vi "1_Main.vi"() -> ()   [LabVIEW 2014]
uses:
  <vilib>/Platform/TimedLoop/XDataNode/timing_clust.ctl
  <vilib>/Platform/TimedLoop/XDataNode/nitl_modes.ctl
  <vilib>/Platform/TimedLoop/XDataNode/wakeup.ctl
  <vilib>/myRIO/Instrument Drivers/Onboard IO/UART/typedef/VISA Configuration.ctl
  <vilib>/myRIO/Instrument Drivers/Onboard IO/DIO/typedefs/DIO Reference.ctl
  <vilib>/myRIO/Common/Instrument Driver Framework/Utilities/typedefs/myRIO Generic Hardware Reference.ctl
  <vilib>/myRIO/Common/Instrument Driver Framework/Utilities/typedefs/Hardware Version Enum.ctl
  <vilib>/myRIO/Common/Instrument Driver Framework/Utilities/typedefs/myRIO v1.0 Reference.ctl
  <vilib>/myRIO/Common/Instrument Driver Framework/Utilities/typedefs/Generic FPGA Reference.ctl
  <vilib>/myRIO/Common/Instrument Driver Framework/myRIO v1.0/DIO/typedefs/DIO Channels List.ctl
  <vilib>/myRIO/Common/Instrument Driver Framework/myRIO v1.0/DIO/typedefs/DIO Channels Enum.ctl
  <vilib>/userdefined/High Color/nirio_resource_hc.ctl
  <vilib>/myRIO/Instrument Drivers/Onboard Devices/Accelerometer/typedefs/Accelerometer Reference.ctl
  <vilib>/myRIO/Common/Instrument Driver Framework/myRIO v1.0/Accelerometer/typedefs/Accelerometer Channels List.ctl
  <vilib>/myRIO/Common/Instrument Driver Framework/myRIO v1.0/Accelerometer/typedefs/Accelerometer Channels Enum.ctl
  <vilib>/myRIO/Common/Instrument Driver Framework/Utilities/vis/Is FPGA Ref Available.vi
  <vilib>/myRIO/Common/Instrument Driver Framework/myRIO v1.0/DIO/vis/myRIO v1.1 Open DIO.vi
  <vilib>/myRIO/Instrument Drivers/Onboard IO/DIO/vis/Write.vi
  <vilib>/myRIO/Common/Instrument Driver Framework/myRIO v1.0/Accelerometer/vis/myRIO v1.1 Open Accelerometer.vi
  <vilib>/myRIO/Instrument Drivers/Onboard Devices/Accelerometer/vis/Read.vi
  <vilib>/myRIO/Common/Instrument Driver Framework/Utilities/vis/Validate Channels.vi
  <vilib>/myRIO/Common/Instrument Driver Framework/myRIO v1.0/DIO/vis/myRIO v1.0 Reserve DIO.vi
  <vilib>/myRIO/Common/Instrument Driver Framework/myRIO v1.0/Accelerometer/vis/myRIO v1.0 Reserve Accelerometer.vi
  <vilib>/myRIO/Common/Instrument Driver Framework/myRIO v1.0/UART/vis/myRIO v1.0 Close UART.vi
  <vilib>/myRIO/Common/Instrument Driver Framework/myRIO v1.0/Resource Manager/vis/myRIO v1.0 Reserve Channel List.vi
  <vilib>/myRIO/Common/Instrument Driver Framework/myRIO v1.0/DIO/vis/myRIO v1.0 Build MUX Configuration DIO.vi
  <vilib>/myRIO/Common/Instrument Driver Framework/myRIO v1.0/Accelerometer/vis/myRIO v1.0 Build MUX Configuration Accelerometer.vi
  <vilib>/myRIO/Common/Instrument Driver Framework/myRIO v1.0/Resource Manager/vis/myRIO v1.0 Reserve Channel.vi
  <vilib>/myRIO/Common/Instrument Driver Framework/myRIO v1.0/Resource Manager/vis/myRIO v1.0 Unreserve Channel.vi
  <vilib>/myRIO/Common/Instrument Driver Framework/myRIO v1.0/Resource Manager/vis/myRIO v1.0 Create Configuration List.vi
  <vilib>/myRIO/Common/Instrument Driver Framework/myRIO v1.0/Resource Manager/vis/myRIO v1.0 Build Mutex Name.vi
  <vilib>/Instr/_visa.llb/VISA Configure Serial Port (Instr).vi
  <vilib>/Utility/VariantDataType/GetNumericInfo.vi
  <vilib>/Utility/error.llb/Error Cluster From Error Code.vi
  <vilib>/myRIO/Common/Instrument Driver Framework/myRIO v1.0/myRIO v1.1 Open.vi
  <vilib>/myRIO/Common/Instrument Driver Framework/Utilities/vis/IO Manager.vi
  <vilib>/myRIO/Common/Instrument Driver Framework/Utilities/vis/Configuration Manager.vi
  <vilib>/myRIO/Common/Instrument Driver Framework/myRIO v1.0/Resource Manager/vis/myRIO v1.0 Configure IO.vi
  <vilib>/myRIO/Common/Instrument Driver Framework/myRIO v1.0/myRIO v1.0 Close.vi
  <vilib>/myRIO/Common/Instrument Driver Framework/myRIO v1.0/DIO/vis/myRIO v1.0 Write DIO.vi
  <vilib>/myRIO/Common/Instrument Driver Framework/myRIO v1.0/Accelerometer/vis/myRIO v1.0 Get Scaling Constant Accelerometer.vi
  <vilib>/myRIO/Common/Instrument Driver Framework/myRIO v1.0/Accelerometer/vis/myRIO v1.0 Read Accelerometer.vi
  <vilib>/myRIO/Common/Instrument Driver Framework/Utilities/vis/FPGA Ref Manager.vi
  <vilib>/myRIO/Common/Instrument Driver Framework/myRIO v1.0/myRIO v1.0 Reset FPGA.vi
  <vilib>/myRIO/Common/Instrument Driver Framework/myRIO v1.0/IRQ/vis/myRIO v1.0 IRQ Info FGV.vi
  <vilib>/myRIO/Common/Instrument Driver Framework/myRIO v1.0/IRQ/vis/myRIO v1.0 Timer IRQ Info FGV.vi
  <vilib>/myRIO/Common/Instrument Driver Framework/myRIO v1.0/IRQ/vis/myRIO v1.0 ISR Agent.vi
  <vilib>/myRIO/Express VI/Onboard IO/UART/UART Express VI.xnode
  <vilib>/platform/TimedLoop/XDataNode/XDataNode.xnode
  <vilib>/myRIO/Express VI/Onboard Devices/LED/LED Express VI.xnode
  <vilib>/myRIO/Instrument Drivers/Onboard IO/DIO/vis/myRIO DIO Open.xnode
  <vilib>/myRIO/Express VI/Onboard Devices/Accelerometer/Accelerometer Express VI.xnode
  <vilib>/myRIO/Instrument Drivers/Onboard Devices/Accelerometer/vis/myRIO Accelerometer Open.xnode
  <vilib>/myRIO/Instrument Drivers/Utilities/Utilities.lvlib
  <vilib>/myRIO/Instrument Drivers/Onboard Devices/Accelerometer/Accelerometer.lvlib
  <vilib>/myRIO/Instrument Drivers/Onboard IO/DIO/DIO.lvlib
  <vilib>/myRIO/Instrument Drivers/Onboard IO/UART/UART.lvlib
  <vilib>/Platform/TimedLoop/XDataNode/XDNodeRunTimeDep.lvlib
panel:
  out "Measured Angle":dbl
  out "Simulation Angle":dbl
  out "Receive Distance":bool
  out "Velocity Display":dbl(graph)
  out "Data File Path":path=path "c:/ni-rt/startup/11_25_14_03:39 AM.csv"
  out "Read Finished Late?":bool
  out "Velocity (cm/s)":dbl(slide) scale=0.0..100.0
  out "match substring":string
  out "Distance (cm)":dbl
  in  "Simulation":bool=TRUE
  in  "PS 14":bool caption="1"
  in  "PS 13":bool caption="1"
  in  "PS 12":bool caption="1"
  in  "PS 11":bool caption="1"
  in  "PS 10":bool caption="1"
  in  "PS 9":bool caption="1"
  in  "PS 8":bool caption="1"
  in  "PS 7":bool caption="1"
  in  "PS 6":bool caption="1"
  in  "PS 5":bool caption="1"
  in  "PS 4":bool caption="1"
  in  "PS 3":bool caption="1"
  in  "PS 2":bool caption="1"
  in  "PS 1":bool caption="1"
  in  "Arm Leg Angle Ratio":dbl(slide)=0.9696969696969697 scale=0.0..2.0
  in  "Ground":dbl(slide)=400.00000000000006 scale=0.0..450.0
  in  "Horizontal Center":dbl(slide)=395.95959595959596 scale=0.0..800.0
  out "Characters Read":string
  out "Mannequin Motion":picture
  out "Joint A":dbl(knob)=7.460836761961528 scale=40.0..-40.0 scale format="%#.1f"
  in  "Scale Factor":dbl(slide)=0.5707070707070707 scale=0.5..1.0
  in  "LED3":bool
  in  "LED2":bool
  in  "LED1":bool
  in  "LED0":bool
  out "Acceleration":T1(graph)={"X-Axis"=0.0625, "Y-Axis"=0.109375, "Z-Axis"=1.0}
  out "error out":errorcluster
  in  "Stop Button":bool
  # "Overview: The myRIO Project template acquires acceleration data from the onboard accelerometer and displays the changes of acceleration values in a waveform chart.\nInstructions:\n1. Check the myRIO target IP Address in the project and make sure the target IP Address is correct. \n2. Run the VI."
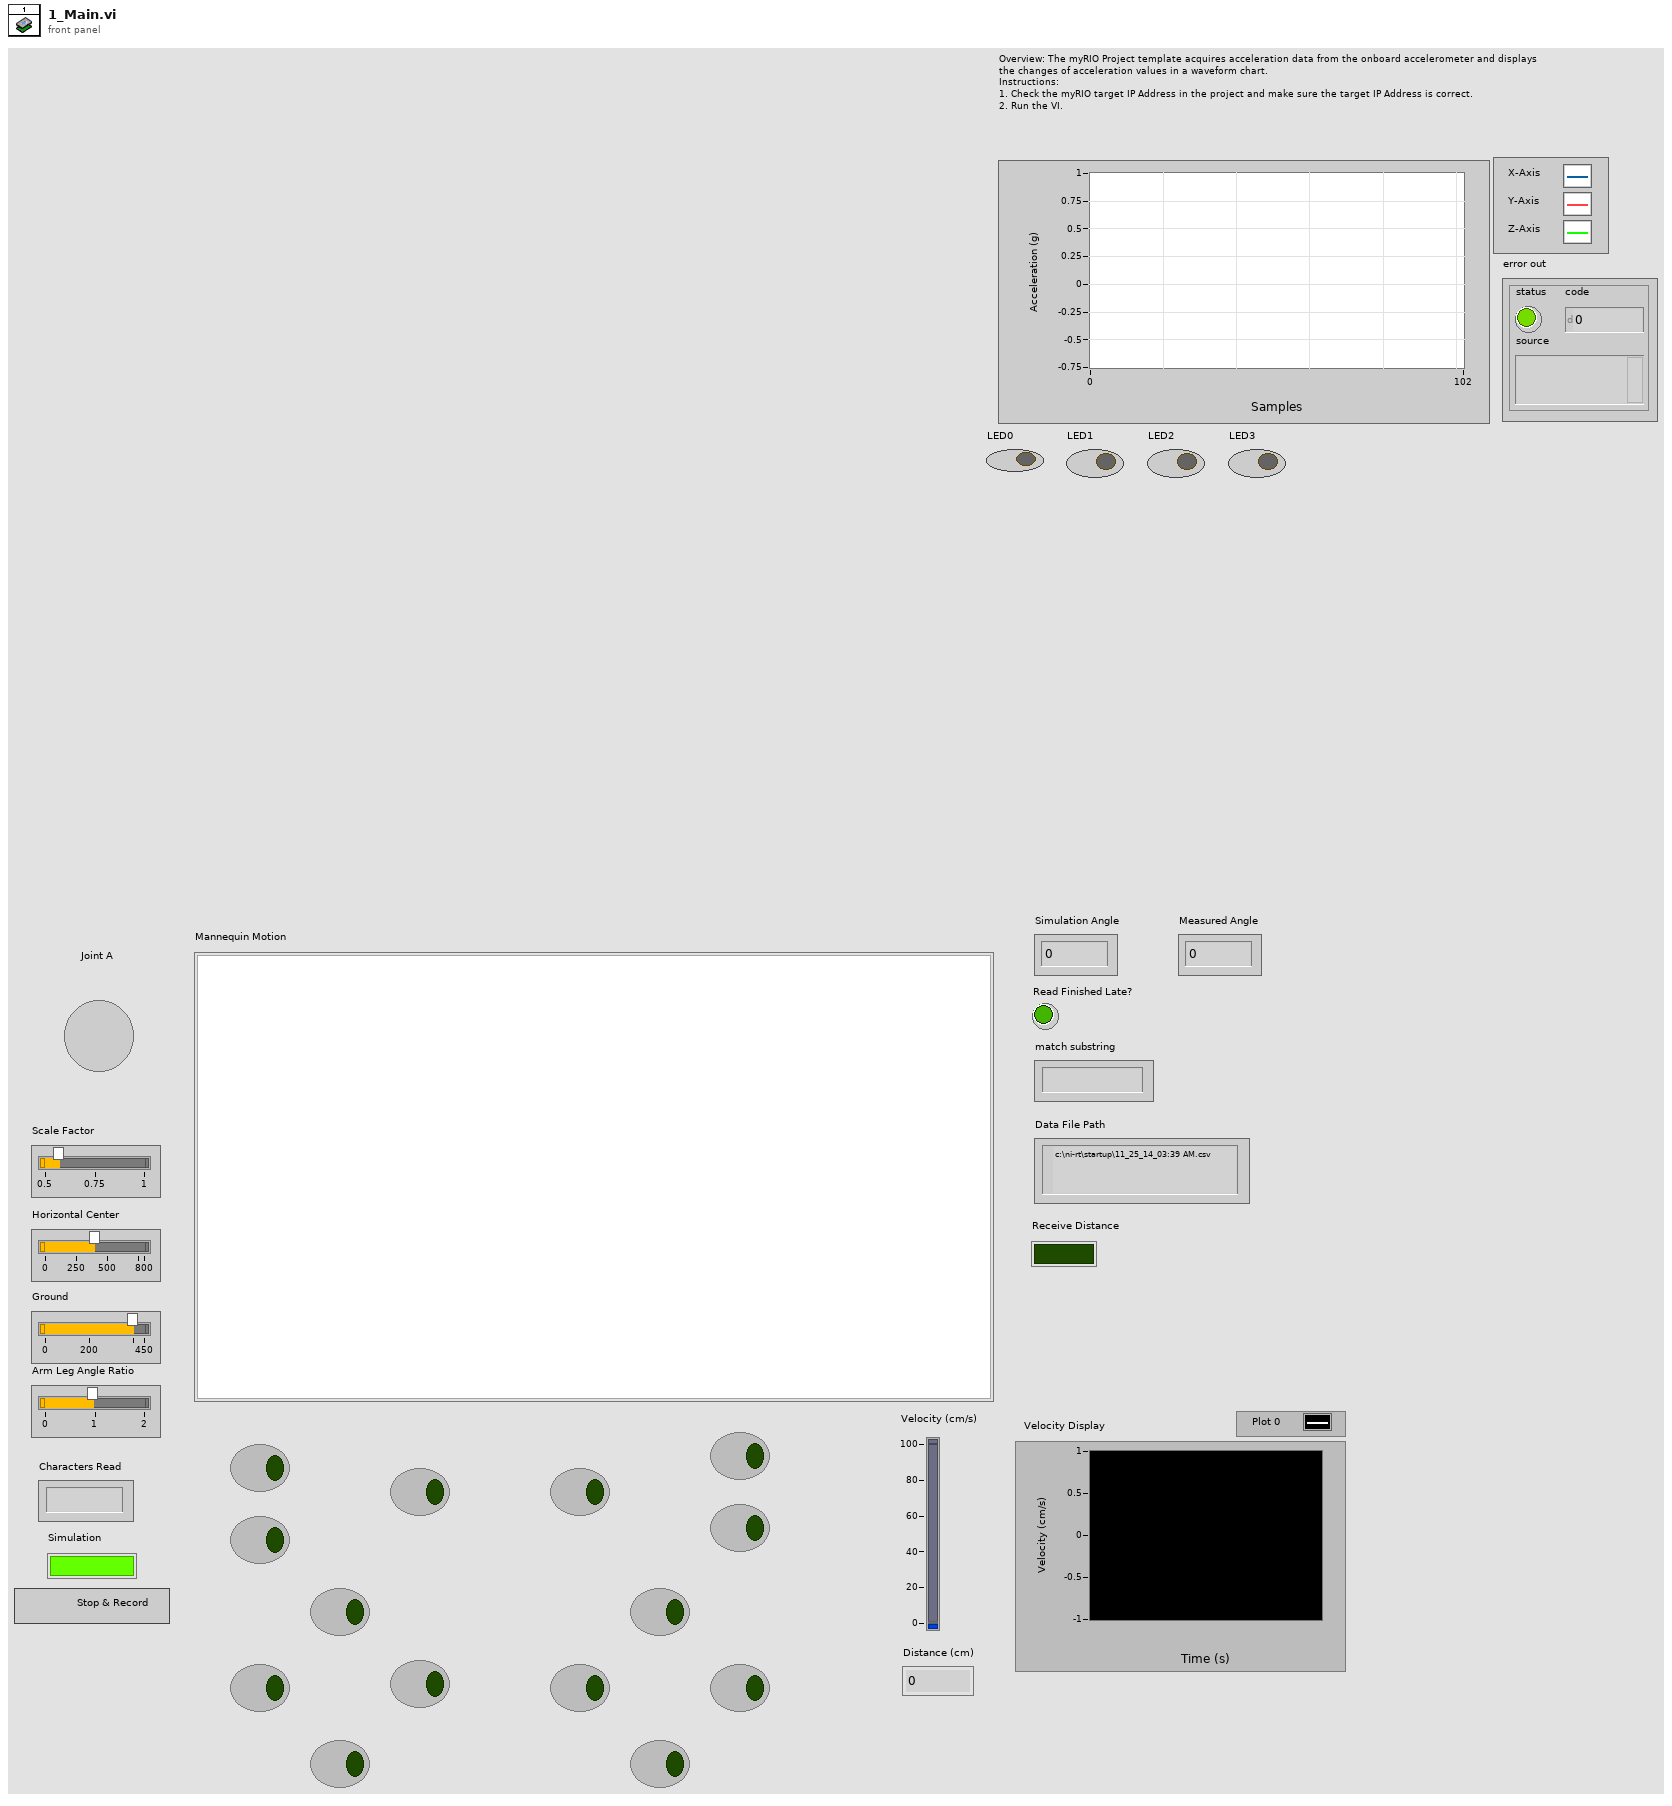
[diagram p1: front panel]
types:
  T1 = cluster{"X-Axis":dbl, "Y-Axis":dbl, "Z-Axis":dbl}
  T2 = typedef "XDNodeRunTimeDep.lvlib/timing_clust.ctl" = cluster{"Expected End [f-1]":u64, "Actual End [f-1]":u64, "Finished Late? [f-1]":bool, "Expected End [i-1]":u64, "Actual End [i-1]":u64, "Finished Late? [i-1]":bool, "Expected Start [i]":u64, "Actual Start [i]":u64, "Expected Start [f]":u64, "Actual Start [f]":u64, "Source Name":string, "Structure Name":string, "Period":i64, "Deadline":i64, "Offset":i64, "Start":i64, "Priority":i32, "Timeout":i32, "Mode":T3, "Wakeup Reason":T4, "Error":errorcluster, "Source Type":string, "Secondary Source Type":string, "Global End Time":u64, "Global Start Time":u64, "Frame Duration":u64, "Iteration Duration":u64, "Assigned CPU":i32, "I/O Scan Engine Mode":u32}
  T3 = typedef "XDNodeRunTimeDep.lvlib/nitl_modes.ctl" = enum32{"No Change", "Process missed periods, maintain original phase", "Discard missed periods, maintain original phase", "Process missed periods, ignore original phase", "Discard missed periods, ignore original phase"}
  T4 = typedef "XDNodeRunTimeDep.lvlib/wakeup.ctl" = enum32{"Normal", "Aborted", "Asynchronous wakeup", "Timing source error", "Timed loop error", "Timeout"}
  T5 = typedef "UART.lvlib/VISA Configuration.ctl" = cluster{"baud rate (9600)":u32, "data bits (8)":u16, "parity (0:none)":enum16{"None", "Odd", "Even", "Mark", "Space"}, "stop bits (10: 1 bit)":u16, "flow control (0:none)":u16, "termination char\n(0xA = '\\n' = LF) ":u8, "Enable Termination\nChar (T)":bool, "timeout (10sec)":u32}
  T6 = cluster{"Width":u16, "Style":enum32{"Solid", "Dash", "Dot", "DashDot", "DashDotDot"}}
  T7 = cluster{"left":i16, "top":i16, "right":i16, "bottom":i16}
  T8 = typedef "DIO.lvlib/DIO Reference.ctl" = cluster{"myRIO Reference":T9, "DIO Channels List":T13}
  T9 = typedef "myRIO Generic Hardware Reference.ctl" = cluster{"myRIO Model":T10, "myRIO Hardware Reference":T11}
  T10 = typedef "Hardware Version Enum.ctl" = enum16{"Unknown", "myRIO-1900", "myRIO-1950"}
  T11 = typedef "myRIO v1.0 Reference.ctl" = cluster{"Generic FPGA Reference":T12, "Allow multiple opens":bool}
  T12 = typedef "Generic FPGA Reference.ctl" = refnum<k20>
  T13 = typedef "DIO Channels List.ctl" = T14[]
  T14 = typedef "DIO Channels Enum.ctl" = enum16{"Not Connected", "C/DIO0", "C/DIO1", "C/DIO2", "C/DIO3", "C/DIO4", "C/DIO5", "C/DIO6", "C/DIO7", "A/DIO0", "A/DIO1", "A/DIO2", "A/DIO3", "A/DIO4", "A/DIO5", "A/DIO6", "A/DIO7", "A/DIO8", "A/DIO9", "A/DIO10", "A/DIO11", "A/DIO12", "A/DIO13", "A/DIO14", "A/DIO15", "B/DIO0", "B/DIO1", "B/DIO2", "B/DIO3", "B/DIO4", "B/DIO5", "B/DIO6", "B/DIO7", "B/DIO8", "B/DIO9", "B/DIO10", "B/DIO11", "B/DIO12", "B/DIO13", "B/DIO14", "B/DIO15", "LED0", "LED1", "LED2", "LED3", "Button0"}
  T15 = typedef "nirio_resource_hc.ctl" = tag
  T16 = typedef "Accelerometer.lvlib/Accelerometer Reference.ctl" = cluster{"myRIO Reference":T9, "Accelerometer Channels List":T17, "LSB Weight":dbl}
  T17 = typedef "Accelerometer Channels List.ctl" = T18[]
  T18 = typedef "Accelerometer Channels Enum.ctl" = enum16{"Not Connected", "X-Axis", "Y-Axis", "Z-Axis"}
  T19 = enum16{"open", "replace", "create", "open or create", "replace or create", "replace or create with confirmation"}
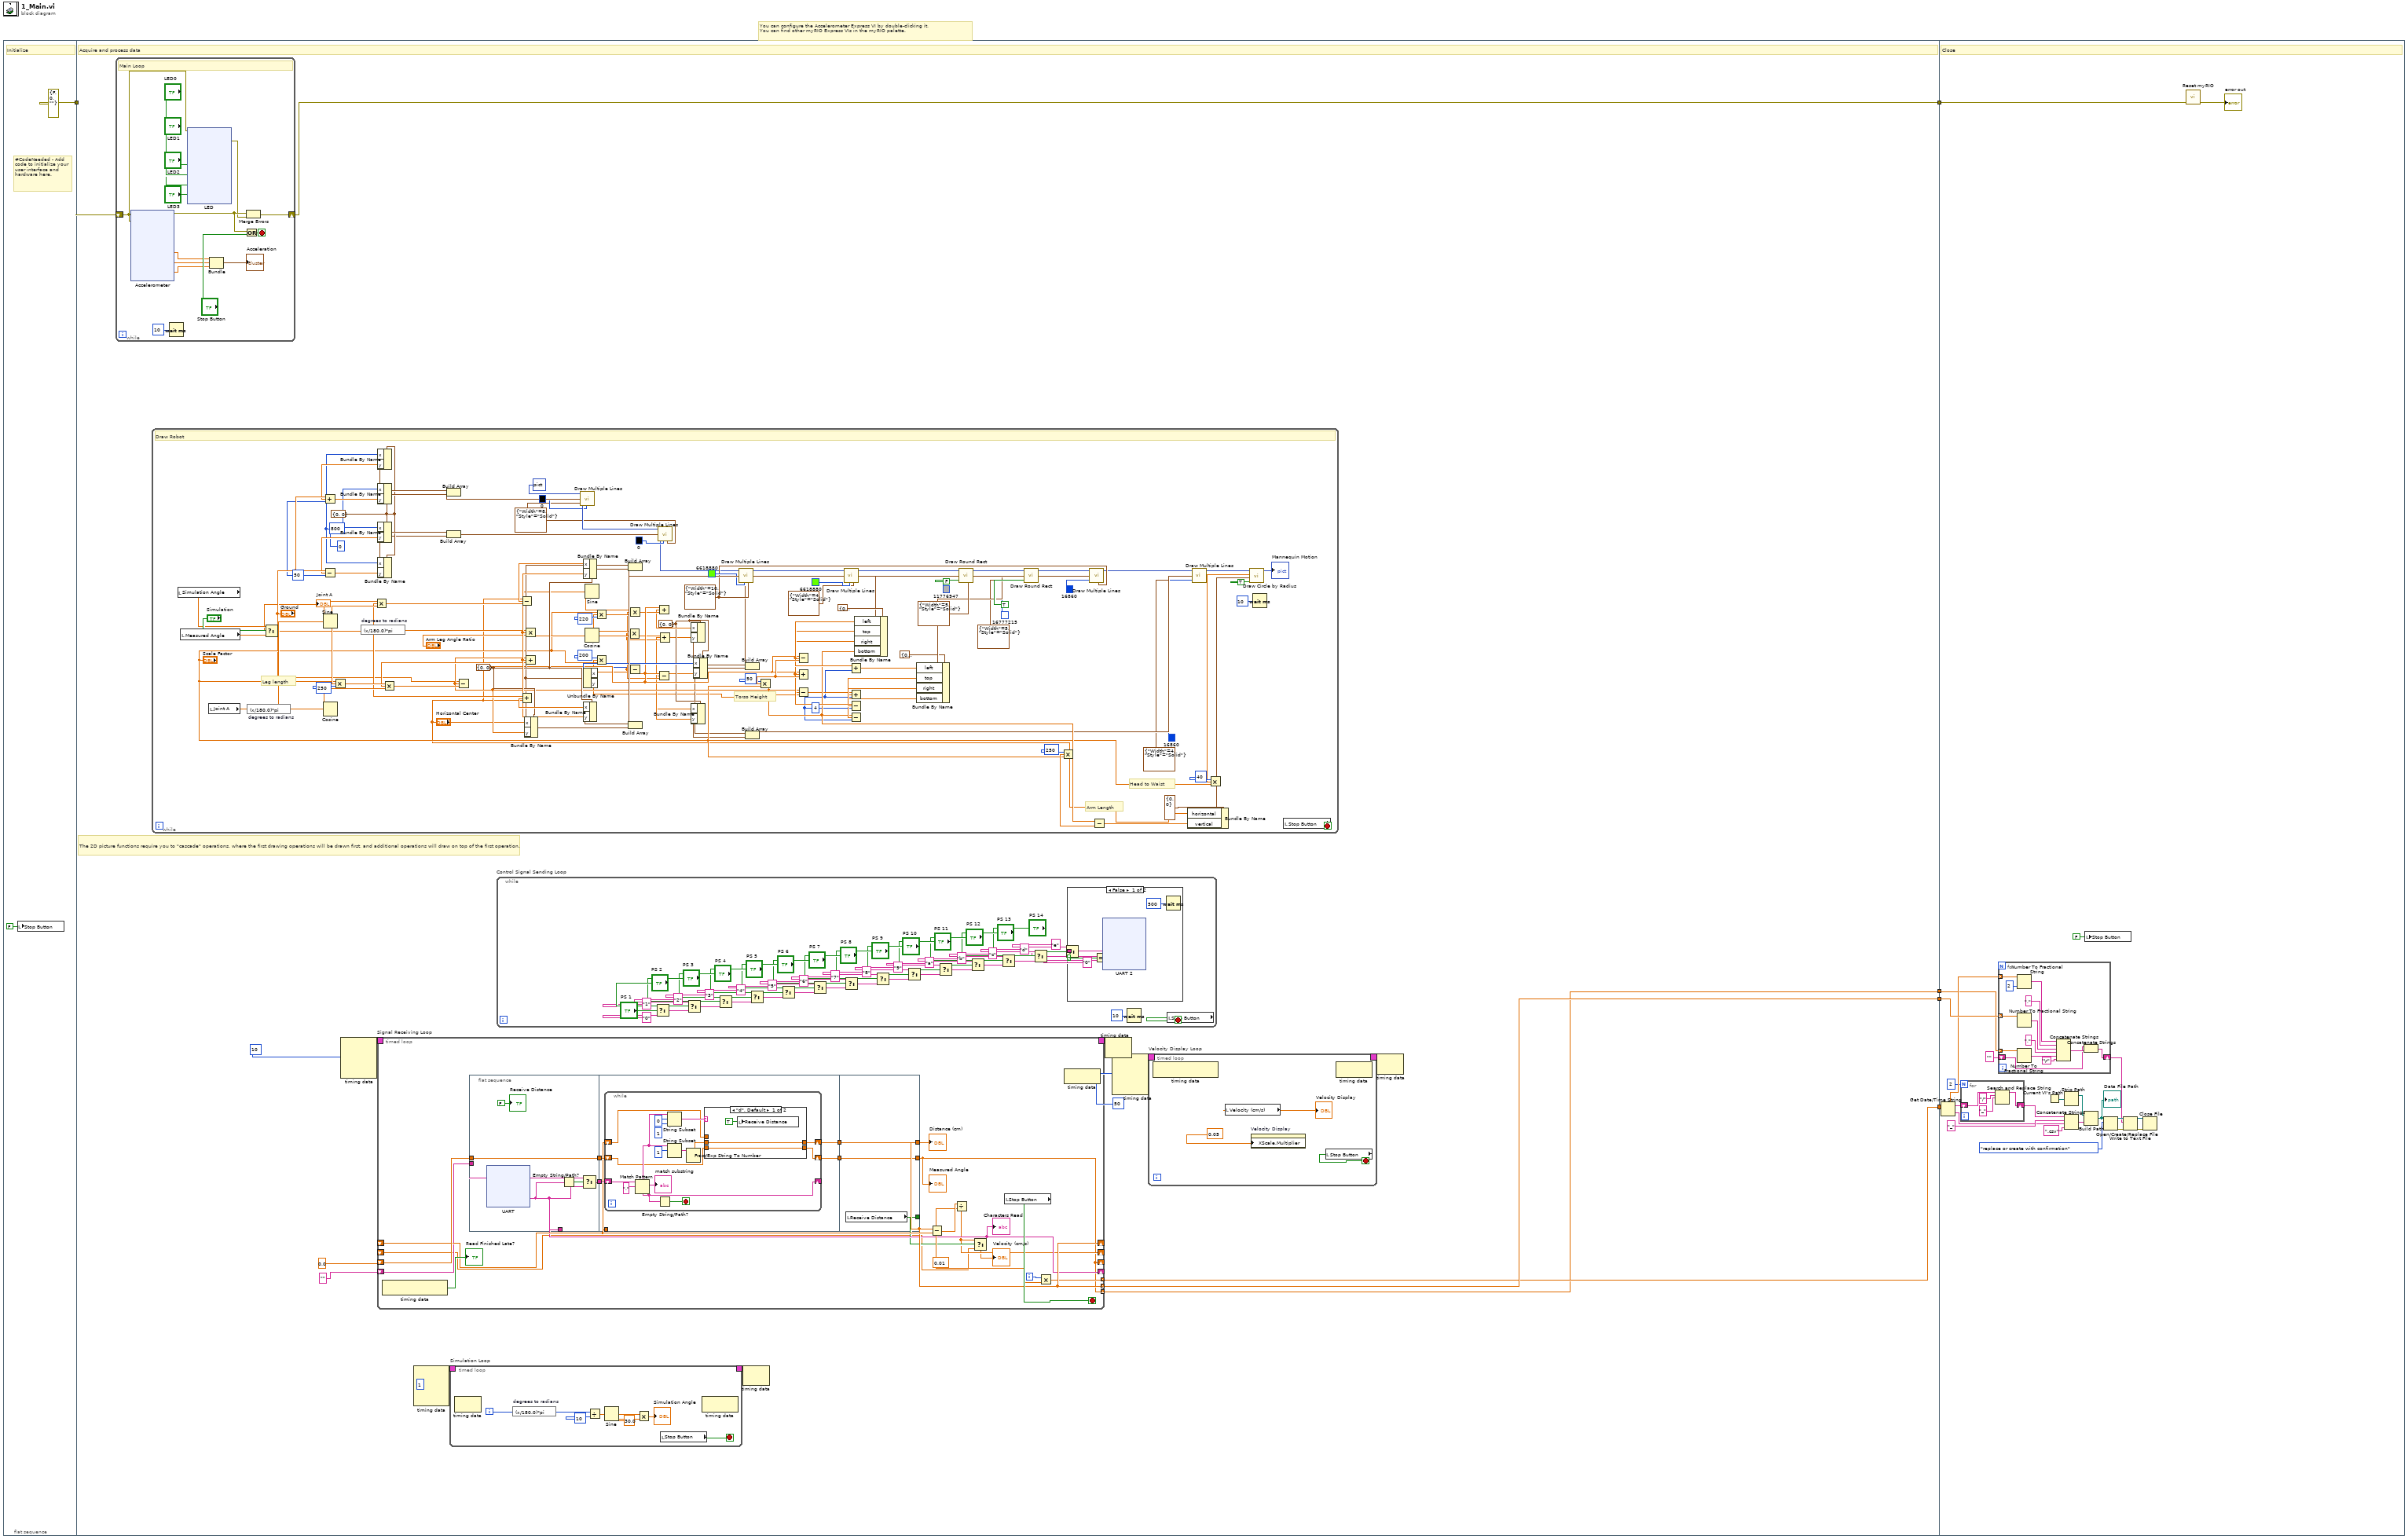
[diagram p0: block diagram]
diagram:
  # "You can configure the Accelerometer Express VI by double-clicking it.\nYou can find other myRIO Express VIs in the myRIO palette."
  n1 = flat-sequence {
    tunnel: [errorcluster {"status"=FALSE, "code"=0, "source"=""} ("error out")] -> w5
    tunnel: w5 -> [w23]
    tunnel: [w22] -> w4
    tunnel: [w16] -> w3
    tunnel: [w15] -> w2
    tunnel: [w14] -> w1
    tunnel: w4 -> [w415]
    tunnel: w3 -> [w406]
    tunnel: w2 -> [w405]
    tunnel: w1 -> [w404]
    frame #0 {
      # "#CodeNeeded - Add code to initialize your user interface and hardware here."
      # "Initialize"
      n2 = local write "Stop Button"(FALSE ("Stop Button")) -> ()
    }
    frame #1 {
      # "The 2D picture functions require you to \"cascade\" operations, where the first drawing operations will be drawn first, and additional operations will draw on top of the first operation."
      # "Acquire and process data"
      n3 = while {
        shift-right: [w301] -> w22
        shift-left: w23 -> [w302]
        stop <- w314 stop-if-true
        # "Main Loop"
        n4 = xnode "Accelerometer"("error in (no error)"=w302) -> ("X-Axis"=w311:dbl, "Y-Axis"=w310:dbl, "Z-Axis"=w309:dbl, "error out"=w304:errorcluster)
        n5 = Wait (ms)(milliseconds to wait=u32 10) -> ()  [unwired: 1 out]
        n6 = xnode "LED"("LED0"="LED0", "LED1"="LED1", "LED2"="LED2", "LED3"="LED3", "error in (no error)"=w302) -> ("error out"=w303:errorcluster)
        n7 = Bundle("X-Axis"=w311, "Y-Axis"=w310, "Z-Axis"=w309) -> (→"Acceleration":T1)  [unwired: 1 in]
        n8 = Or(x=w304, y="Stop Button") -> (x .or. y?=w314:bool)
        n9 = Merge Errors(w304, w303) -> (w301:errorcluster)
      }
      n10 = while {
        stop <- w299 stop-if-true
        w196 = T6 {"Width"=8, "Style"=enum."Solid"} ("pen")
        w214 = i16 0 ("x")
        w195 = i16 800 ("x")
        w220 = i16 50 ("x")
        w212 = cluster{"x":i16, "y":i16} {"x"=0, "y"=0}
        w230 = cluster{"x":i16, "y":i16} {"x"=0, "y"=0}
        w253 = i16 4 ("x")
        w283 = cluster{"x":i16, "y":i16} {"x"=0, "y"=0}
        w264 = T6 {"Width"=10, "Style"=enum."Solid"} ("pen")
        # "Head to Waist"
        # "Arm Length"
        # "Leg length"
        # "Torso Height"
        # "Draw Robot"
        n11 = local read "Simulation Angle"() -> (w193:dbl)
        n12 = local read "Measured Angle"() -> (w192:dbl)
        n13 = local read "Joint A"() -> (w293:dbl)
        n14 = expression code="(x/180.0)*pi" "degrees to radians"(w293) -> (w291:dbl)
        n15 = Select(t=w193, s="Simulation", f=w192) -> (s? t:f=w191:dbl)
        "Joint A" <- w191
        n16 = Add(x="Ground", y=w220) -> (x+y=w219:dbl)
        n17 = Subtract(x="Ground", y=w220) -> (x-y=w215:dbl)
        n18 = Sine(x=w291) -> (sin(x)=w290:dbl)
        n19 = Cosine(x=w291) -> (cos(x)=w288:dbl)
        n20 = Multiply(x="Scale Factor", y=i16 250 ("x")) -> (x*y=w289:dbl)
        n21 = expression code="(x/180.0)*pi" "degrees to radians"(w191) -> (w243:dbl)
        n22 = Multiply(x=w290, y=w289) -> (x*y=w273:dbl)
        n23 = Bundle By Name(cluster=w212, "x"=w195, "y"=w219) -> (w218:cluster{"x":i16, "y":i16})
        n24 = Bundle By Name(cluster=w212, "x"=w214, "y"=w219) -> (w217:cluster{"x":i16, "y":i16})
        n25 = Bundle By Name(cluster=w212, "x"=w214, "y"=w215) -> (w213:cluster{"x":i16, "y":i16})
        n26 = Bundle By Name(cluster=w212, "x"=w195, "y"=w215) -> (w211:cluster{"x":i16, "y":i16})
        n27 = Multiply(x=w289, y=w288) -> (x*y=w263:dbl)
        n28 = Build Array(w218, w217) -> (w216:cluster{"x":i16, "y":i16}[])
        n29 = Build Array(w213, w211) -> (w210:cluster{"x":i16, "y":i16}[])
        n30 = Subtract(x="Ground", y=w263) -> (x-y=w255:dbl)
        n31 = Subtract(x="Horizontal Center", y=w273) -> (x-y=w286:dbl)
        n32 = Add(x=w273, y="Horizontal Center") -> (x+y=w287:dbl)
        n33 = Multiply(x=w243, y="Arm Leg Angle Ratio") -> (x*y=w241:dbl)
        n34 = Add(x=w255, y=w263) -> (x+y=w285:dbl)
        n35 = Bundle By Name(cluster=w283, "x"="Horizontal Center", "y"=w255) -> (w246:cluster{"x":i16, "y":i16})
        n36 = call <vilib>:"Draw Multiple Lines.vi"("picture"=picture data[5B], "line endpoints"=w216, "color(black)"=u32 0, "pen"=w196) -> ("new picture"=w208:picture)  [unwired: 5 in]
        n37 = Bundle By Name(cluster=w283, "x"=w286, "y"=w285) -> (w272:cluster{"x":i16, "y":i16})
        n38 = Bundle By Name(cluster=w283, "x"=w287, "y"=w285) -> (w284:cluster{"x":i16, "y":i16})
        n39 = Unbundle By Name(w246) -> ("x"=w244:i16, "y"=w205:i16)
        n40 = Sine(x=w241) -> (sin(x)=w237:dbl)
        n41 = Cosine(x=w241) -> (cos(x)=w238:dbl)
        n42 = Multiply(x="Scale Factor", y=i16 220 ("x")) -> (x*y=w236:dbl)
        n43 = Multiply(x=i16 200, y="Scale Factor") -> (x*y=w204:dbl)
        n44 = Multiply(x=w236, y=w238) -> (x*y=w233:dbl)
        n45 = Multiply(x=w237, y=w236) -> (x*y=w234:dbl)
        n46 = Subtract(x=w205, y=w204) -> (x-y=w203:dbl)
        n47 = Build Array(w246, w272) -> (w271:cluster{"x":i16, "y":i16}[])
        n48 = Build Array(w284, w246) -> (w282:cluster{"x":i16, "y":i16}[])
        n49 = Add(x="Horizontal Center", y=w234) -> (x+y=w232:dbl)
        n50 = Subtract(x="Horizontal Center", y=w234) -> (x-y=w228:dbl)
        n51 = Add(x=w203, y=w233) -> (x+y=w229:dbl)
        n52 = call <vilib>:"Draw Multiple Lines.vi"("picture"=w208, "line endpoints"=w210, "color(black)"=u32 0, "pen"=w196) -> ("new picture"=w200:picture)  [unwired: 5 in]
        n53 = Bundle By Name(cluster=w230, "x"=w232, "y"=w229) -> (w247:cluster{"x":i16, "y":i16})
        n54 = Bundle By Name(cluster=w230, "x"=w228, "y"=w229) -> (w227:cluster{"x":i16, "y":i16})
        n55 = Bundle By Name(cluster=w230, "x"=w244, "y"=w203) -> (w226:cluster{"x":i16, "y":i16})
        n56 = call <vilib>:"Draw Multiple Lines.vi"("picture"=w200, "line endpoints"=w271, "color(black)"=u32 6618880, "pen"=w264) -> ("new picture"=w199:picture)  [unwired: 5 in]
        n57 = Build Array(w247, w226) -> (w245:cluster{"x":i16, "y":i16}[])
        n58 = Build Array(w226, w227) -> (w225:cluster{"x":i16, "y":i16}[])
        n59 = Multiply(x=i16 50, y="Scale Factor") -> (x*y=w296:dbl)
        n60 = Subtract(x="Horizontal Center", y=w296) -> (x-y=w260:dbl)
        n61 = Add(x="Horizontal Center", y=w296) -> (x+y=w258:dbl)
        n62 = Subtract(x=w255, y=w204) -> (x-y=w254:dbl)
        n63 = call <vilib>:"Draw Multiple Lines.vi"("picture"=w199, "line endpoints"=w245, "color(black)"=u32 6618880, "pen"=T6 {"Width"=4, "Style"=enum."Solid"}) -> ("new picture"=w231:picture)  [unwired: 5 in]
        n64 = Add(x=w260, y=w253) -> (x+y=w259:dbl)
        n65 = Add(x=w254, y=w253) -> (x+y=w248:dbl)
        n66 = Subtract(x=w258, y=w253) -> (x-y=w257:dbl)
        n67 = Subtract(x=w255, y=w253) -> (x-y=w256:dbl)
        n68 = Bundle By Name(cluster=T7 {"left"=0, "top"=0, "right"=0, "bottom"=0} ("rect"), "left"=w260, "top"=w254, "right"=w258, "bottom"=w255) -> (w297:T7)
        n69 = Bundle By Name(cluster=T7 {"left"=0, "top"=0, "right"=0, "bottom"=0} ("rect"), "left"=w259, "top"=w248, "right"=w257, "bottom"=w256) -> (w252:T7)
        n70 = call <vilib>:"Draw Round Rect.vi"("picture"=w231, "rect"=w297, "fill?(F)"=FALSE, "color(black)"=u32 11776947, "pen"=T6 {"Width"=5, "Style"=enum."Solid"}) -> ("new picture"=w262:picture)  [unwired: 4 in]
        n71 = call <vilib>:"Draw Round Rect.vi"("picture"=w262, "rect"=w252, "fill?(F)"=TRUE, "color(black)"=u32 16777215, "pen"=T6 {"Width"=5, "Style"=enum."Solid"}) -> ("new picture"=w198:picture)  [unwired: 4 in]
        n72 = Multiply(x=i16 250, y="Scale Factor") -> (x*y=w266:dbl)
        n73 = call <vilib>:"Draw Multiple Lines.vi"("picture"=w198, "line endpoints"=w282, "color(black)"=u32 16860, "pen"=w264) -> ("new picture"=w197:picture)  [unwired: 5 in]
        n74 = Subtract(x=w255, y=w266) -> (x-y=w265:dbl)
        n75 = Bundle By Name(cluster=cluster{"horizontal":i16, "vertical":i16} {"horizontal"=0, "vertical"=0} ("pixel center"), "horizontal"="Horizontal Center", "vertical"=w265) -> (w279:cluster{"horizontal":i16, "vertical":i16})
        n76 = call <vilib>:"Draw Multiple Lines.vi"("picture"=w197, "line endpoints"=w225, "color(black)"=u32 16860, "pen"=T6 {"Width"=4, "Style"=enum."Solid"}) -> ("new picture"=w222:picture)  [unwired: 5 in]
        n77 = Multiply(x=i16 40 ("radius"), y="Scale Factor") -> (x*y=w274:dbl)
        n78 = call <vilib>:"Draw Circle by Radius.vi"("fill?(F)"=TRUE, "pixel center"=w279, "radius"=w274, "picture"=w222) -> ("new picture"=→"Mannequin Motion":picture)  [unwired: 7 in]
        n79 = Wait (ms)(milliseconds to wait=u32 10) -> ()  [unwired: 1 out]
        n80 = local read "Stop Button"() -> (w299:bool)
      }
      n81 = node-c288(i64 10 ("Period")) -> (w19:T2)  [unwired: 3 in]
      n82 = timed-loop "Signal Receiving Loop" {
        shift-right: [w54] -> _
        shift-left: "" ("Characters Read") -> [w55]
        shift-right: [w47] -> _
        shift-left: 0.0 -> [w65]
        shift-right: [w62] -> _
        shift-left: _ -> [w63]
        timing: w19 -> [_]
        timing-out: [_] -> w18
        tunnel: [w62] -> w16 mode=indexing
        tunnel: [w58] -> w15 mode=indexing
        tunnel: [w47] -> w14 mode=indexing
        shift-right: [w50] -> _
        shift-left: _ -> [w48]
        i -> [w60]
        stop <- w66 stop-if-true
        w59 = 0.01 ("y")
        n83 = node-c288() -> (→"Read Finished Late?":bool)  [unwired: 1 in]
        n84 = flat-sequence {
          tunnel: w65 -> [w72]
          tunnel: [w69] -> w57
          tunnel: [w72] -> w56
          tunnel: w55 -> [w70]
          tunnel: [w68] -> w54
          tunnel: w63 -> [w91]
          tunnel: w57 -> [w93]
          tunnel: w56 -> [w92]
          tunnel: [w94] -> w53
          tunnel: [w90] -> w52
          tunnel: [w117] -> w62
          tunnel: [w118] -> w47
          tunnel: w53 -> [w118]
          tunnel: w52 -> [w117]
          tunnel: [w116] -> w51
          frame #0 {
            n85 = xnode "UART"() -> ("Characters Read"=w68:string)  [unwired: 1 in, 1 out]
            n86 = Empty String/Path?(string/path=w68) -> (empty?=w71:bool)
            n87 = Select(t=w70, s=w71, f=w68) -> (s? t:f=w69:string)
            "Receive Distance" <- FALSE ("Receive Distance")
          }
          frame #1 {
            n88 = while {
              shift-right: [w99] -> _
              shift-left: w93 -> [w101]
              shift-right: [w102] -> w94
              shift-left: w92 -> [w96]
              shift-right: [w98] -> w90
              shift-left: w91 -> [w95]
              stop <- w100 stop-if-true
              n89 = Match Pattern(string=w101, regular expression=",") -> (before substring=w103:string, match substring=→"match substring":string, after substring=w99:string)  [unwired: 2 out]
              n90 = Empty String/Path?(string/path=w99) -> (empty?=w100:bool)
              n91 = String Subset(string=w103, offset (0)=0, length (rest)=1 ("length (rest)")) -> (substring=w108:string)
              n92 = String Subset(string=w103, offset (0)=1) -> (substring=w107:string)  [unwired: 1 in]
              n93 = Fract/Exp String To Number(string=w107) -> (number=w109:dbl)  [unwired: 3 in, 1 out]
              n94 = case shown="\"d\", Default" w108 {
                tunnel: w109 -> [w113 w115]
                tunnel: [w112 w115] -> w102
                tunnel: [w113 w114] -> w98
                tunnel: w95 -> [_ w114]
                tunnel: w96 -> [w112 _]
                frame "d", Default {
                  n95 = local write "Receive Distance"(TRUE ("Receive Distance")) -> ()
                }
                frame "a" {
                }
              }
            }
          }
          frame #2 {
            n96 = local read "Receive Distance"() -> (w116:bool)
          }
        }
        n97 = Subtract(x=w62, y=w63) -> (x-y=w61:dbl)
        n98 = Divide(x=w61, y=w59) -> (x/y=w50:dbl)
        n99 = Select(t=w50, s=w51, f=w48) -> (s? t:f=→"Velocity (cm/s)":dbl)
        n100 = local read "Stop Button"() -> (w66:bool)
        n101 = Multiply(x=w60, y=w59) -> (x*y=w58:dbl)
        n102 = node-c288() -> ()  [unwired: 1 in, 1 out]
        "Characters Read" <- w54
        "Distance (cm)" <- w62
        "Measured Angle" <- w47
      }
      n103 = node-c288(i64 1 ("Period")) -> (w10:T2)  [unwired: 3 in]
      n104 = timed-loop "Simulation Loop" {
        timing: w10 -> [_]
        timing-out: [_] -> w9
        i -> [w31]
        stop <- w25 stop-if-true
        n105 = node-c288() -> ()  [unwired: 1 in, 1 out]
        n106 = expression code="(x/180.0)*pi" "degrees to radians"(w31) -> (w29:i32)
        n107 = Divide(x=w29, y=10) -> (x/y=w28:dbl)
        n108 = Sine(x=w28) -> (sin(x)=w26:dbl)
        n109 = Multiply(x=w26, y=30.0) -> (x*y=→"Simulation Angle":dbl)
        n110 = local read "Stop Button"() -> (w25:bool)
        n111 = node-c288() -> ()  [unwired: 1 in, 1 out]
      }
      n112 = while "Control Signal Sending Loop" {
        stop <- w163 stop-if-true
        n113 = Select(t="1" ("Characters to Write"), s="PS 1", f="0" ("Characters to Write")) -> (s? t:f=w170:string)
        n114 = Select(t="2" ("Characters to Write"), s="PS 2", f=w170) -> (s? t:f=w154:string)
        n115 = Select(t="3" ("Characters to Write"), s="PS 3", f=w154) -> (s? t:f=w153:string)
        n116 = Select(t="4" ("Characters to Write"), s="PS 4", f=w153) -> (s? t:f=w152:string)
        n117 = Select(t="5" ("Characters to Write"), s="PS 5", f=w152) -> (s? t:f=w151:string)
        n118 = Select(t="6" ("Characters to Write"), s="PS 6", f=w151) -> (s? t:f=w134:string)
        n119 = Select(t="7" ("Characters to Write"), s="PS 7", f=w134) -> (s? t:f=w133:string)
        n120 = Select(t="8" ("Characters to Write"), s="PS 8", f=w133) -> (s? t:f=w132:string)
        n121 = Select(t="9" ("Characters to Write"), s="PS 9", f=w132) -> (s? t:f=w131:string)
        n122 = Select(t="a" ("Characters to Write"), s="PS 10", f=w131) -> (s? t:f=w130:string)
        n123 = Select(t="b" ("Characters to Write"), s="PS 11", f=w130) -> (s? t:f=w129:string)
        n124 = Select(t="c" ("Characters to Write"), s="PS 12", f=w129) -> (s? t:f=w128:string)
        n125 = Select(t="d" ("Characters to Write"), s="PS 13", f=w128) -> (s? t:f=w127:string)
        n126 = Select(t="e" ("Characters to Write"), s="PS 14", f=w127) -> (s? t:f=w126:string)
        n127 = Equal?(x=w126, y="0" ("Characters to Write")) -> (x = y?=w172:bool)
        n128 = case shown="False" w172 {
          tunnel: w126 -> [w174 _]
          frame False {
            n129 = xnode "UART 2"("Characters to Write"=w174) -> ()  [unwired: 1 in, 2 out]
            n130 = Wait (ms)(milliseconds to wait=u32 500) -> ()  [unwired: 1 out]
          }
          frame True {
          }
        }
        n131 = Wait (ms)(milliseconds to wait=u32 10) -> ()  [unwired: 1 out]
        n132 = local read "Stop Button"() -> (w163:bool)
      }
      n133 = node-c288(w9) -> ()  [unwired: 1 out]
      n134 = node-c288(w18) -> ()  [unwired: 1 out]
      n135 = node-c288(i64 50 ("Period")) -> (w13:T2)  [unwired: 3 in]
      n136 = timed-loop "Velocity Display Loop" {
        timing: w13 -> [_]
        timing-out: [_] -> w12
        stop <- w40 stop-if-true
        n137 = node-c288() -> ()  [unwired: 1 in, 1 out]
        n138 = local read "Velocity (cm/s)"() -> (→"Velocity Display":dbl)
        n139 = property on="Velocity Display" class="WFChart (strict)"("XScale.Multiplier"=0.05 ("y")) -> ()  [unwired: 2 in, 2 out]
        n140 = local read "Stop Button"() -> (w40:bool)
        n141 = node-c288() -> ()  [unwired: 1 in, 1 out]
      }
      n142 = node-c288(w12) -> ()  [unwired: 1 out]
    }
    frame #2 {
      # "Close"
      n143 = Get Date/Time String() -> (date string=w401:string, time string=w397:string)  [unwired: 3 in]
      n144 = for {
        N: 2 -> [_]
        shift-right: [w417] -> w399
        shift-left: w401 -> [w416]
        n145 = Search and Replace String(input string=w416, search string="/", replace string="_" ("replace string (\"\")")) -> (result string=w417:string)  [unwired: 5 in, 3 out]
      }
      n146 = for "Data Recording" {
        shift-right: [w427] -> w407
        shift-left: "" -> [w426]
        tunnel: w406 -> [w425] mode=indexing
        tunnel: w405 -> [w422] mode=indexing
        tunnel: w404 -> [w421] mode=indexing
        n147 = Number To Fractional String(number=w422, precision (6)=i16 2) -> (F-format string=w424:string)  [unwired: 2 in]
        n148 = Number To Fractional String(number=w425) -> (F-format string=w430:string)  [unwired: 3 in]
        n149 = Number To Fractional String(number=w421) -> (F-format string=w432:string)  [unwired: 3 in]
        n150 = Concatenate Strings(w424, "," ("string"), w430, "," ("string"), w432, "\r") -> (w428:string)
        n151 = Concatenate Strings(w426, w428) -> (w427:string)
      }
      n152 = Current VI's Path() -> (path=w403:path)
      n153 = Strip Path(path=w403) -> (stripped path=w402:path)  [unwired: 1 out]
      n154 = Concatenate Strings(w399, "_" ("replace string (\"\")"), w397, ".csv" ("replace string (\"\")")) -> (w396:string)
      n155 = Build Path(base path=w402, name or relative path=w396) -> (appended path=w394:path)
      "Data File Path" <- w394
      n156 = local write "Stop Button"(FALSE ("Stop Button")) -> ()
      n157 = Open/Create/Replace File(file path (use dialog)=w394, operation (0:open)=T19."replace or create with confirmation") -> (refnum out=w411:refnum<file>, error out=w410:errorcluster)  [unwired: 4 in, 1 out]
      n158 = Write to Text File(file (use dialog)=w411, text=w407, error in=w410) -> (refnum out=w409:refnum<file>, error out=w408:errorcluster)  [unwired: 1 in, 1 out]
      n159 = Close File(refnum=w409, error in=w408) -> ()  [unwired: 2 out]
      n160 = call <vilib>:"Reset myRIO.vi"("error in (no error)"=w415) -> ("error out"=→"error out":errorcluster)  [unwired: 10 in]
    }
  }
